vi "Construct Event Source Filter.vi"(6 "Exclude?(F)":bool, 8 "error in (no error)":errorcluster, 9 "Ignore Case?":bool, 10 "Exact Match?":bool, 11 "Source ID":string) -> (0 "error out":errorcluster, 3 "Compound Filter out":refnum<class "Event Source Filter.lvclass">)   [LabVIEW 2017, in "Event Source Filter.lvclass"]
uses:
  Event Source Filter.lvclass
  Event Source Filter.lvclass/Event Source Filter.ctl
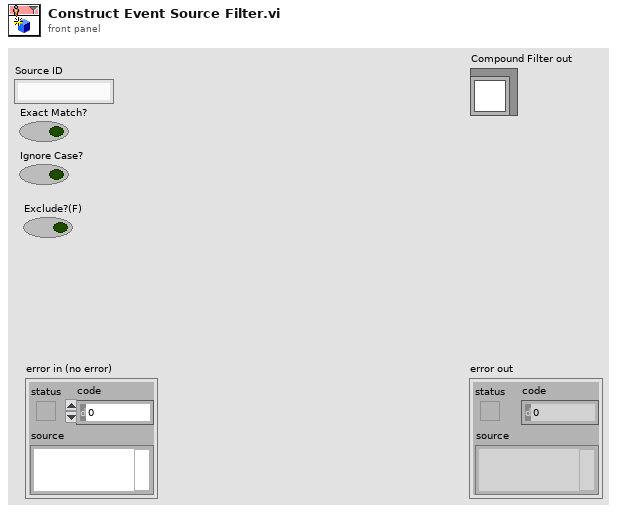
[diagram p1: front panel]
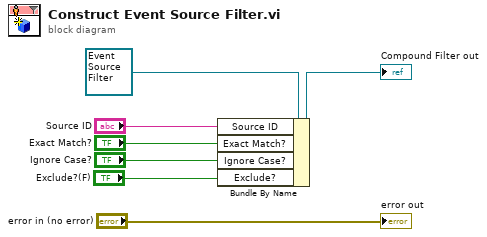
[diagram p0: block diagram]
diagram:
  n1 = Bundle By Name(cluster=refnum<class "Event Source Filter.lvclass"> refnum ("Compound Filter in"), "Source ID"="Source ID", "Exact Match?"="Exact Match?", "Ignore Case?"="Ignore Case?", "Exclude?"="Exclude?(F)") -> (→"Compound Filter out":refnum<class "Event Source Filter.lvclass">)
  "error out" <- "error in (no error)"
